vi "Dispose.vi"(8 "error in (no error)":errorcluster, 11 "Pub Sub Event Channel in":refnum<class "Pub Sub Event Channel.lvclass">) -> (0 "error out":errorcluster, 3 "Pub Sub Event Channel in 2":refnum<class "Pub Sub Event Channel.lvclass">)   [LabVIEW 2020, in "Actor Pub Sub Channels.lvlib" / "Pub Sub Event Channel.lvclass"]
uses:
  Pub Sub Event Channel.lvclass
  Pub Sub Event Channel.lvclass/Pub Sub Event Channel.ctl
  Pub Sub Message Channel/Pub Sub Message Channel.lvclass
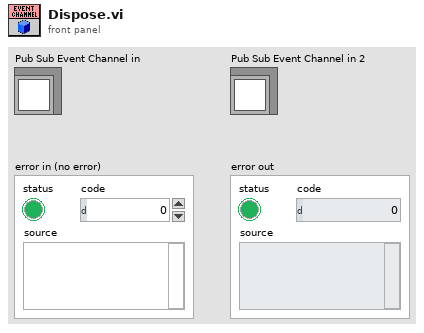
[diagram p1: front panel]
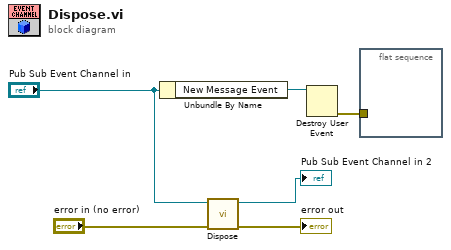
[diagram p0: block diagram]
diagram:
  n1 = Unbundle By Name("Pub Sub Event Channel in") -> ("New Message Event"=w2:refnum<user-event>)
  n2 = call-parent "Dispose.vi"("error in (no error)"="error in (no error)", "Pub Sub Message Channel in"="Pub Sub Event Channel in") -> ("error out"=→"error out":errorcluster, "Pub Sub Message Channel in 2"=→"Pub Sub Event Channel in 2":refnum<class "Pub Sub Event Channel.lvclass">)  [unwired: 8 in]
  n3 = Destroy User Event(user event=w2) -> (error out=w1:errorcluster)  [unwired: 1 in]
  n4 = flat-sequence {
    tunnel: w1 -> [_]
    frame #0 {
    }
  }
